vi "Agilent Source and Measure.vi"() -> ()   [LabVIEW 2021]
doc: "Configures the power supply's output range on a channel, configures the DC voltage level, channel appears at the output connector and takes a measurement on the output signal and returns the measured value."
uses:
  <instrlib>/Agilent 3446X Series/Public/Data/Read (Single Point).vi
  <instrlib>/Agilent N6700 Series/Agilent N6700 Series.lvlib
  <instrlib>/Agilent 3446X Series/Agilent 3446X Series.lvlib
panel:
  in  "error in":errorcluster {"code" format="%.0x"}
  out "error out":errorcluster {"code" format="%.0x"}
  out "DMM Voltage Measurement":dbl
  in  "Manual Range":dbl=1.0
  in  "Agilent DMM":refnum<visa-resource-name>
  in  "Absolute Resolution":dbl=1e-06
  in  "Measurement Function":i32(ring)=10 items=["Continuity", "Current AC", "Current DC", "Diode", "Frequency", "Resistance 4-wire", "Period", "Resistance 2-wire", "Temperature", "Voltage AC", "Voltage DC", "Voltage DC Ratio", "Capacitance"]
  in  "Limit":dbl=1.0 format="%^.3e"
  in  "Behavior":i32(ring) items=["Regulatory Limit", "Trip Limit"]
  out "SMU Voltage Measurement":dbl format="%^.3e"
  in  "Voltage Level":dbl=5.0 format="%^.3e"
  in  "Voltage Range":dbl=10.0 format="%^.3e"
  in  "Channel Name":string="1"
  in  "Agilent SMU":refnum<visa-resource-name>
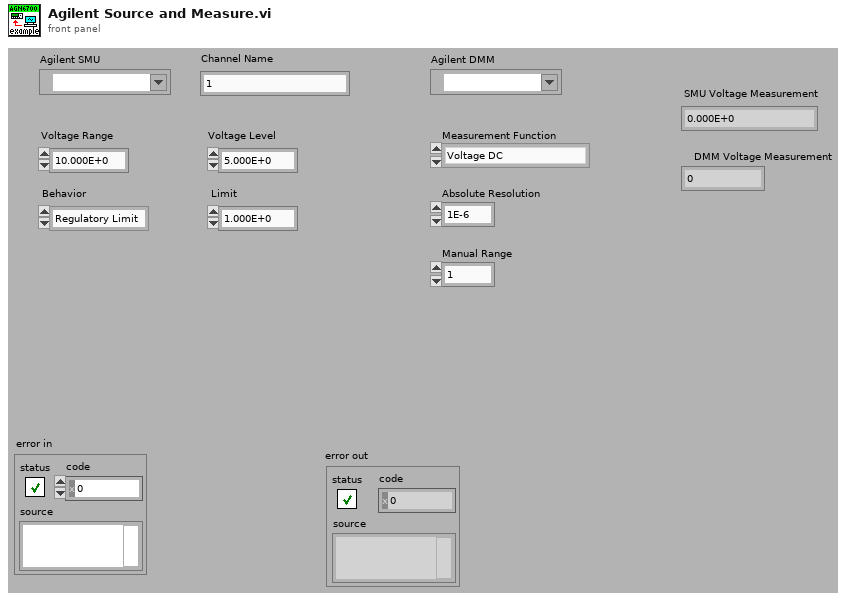
[diagram p1: front panel]
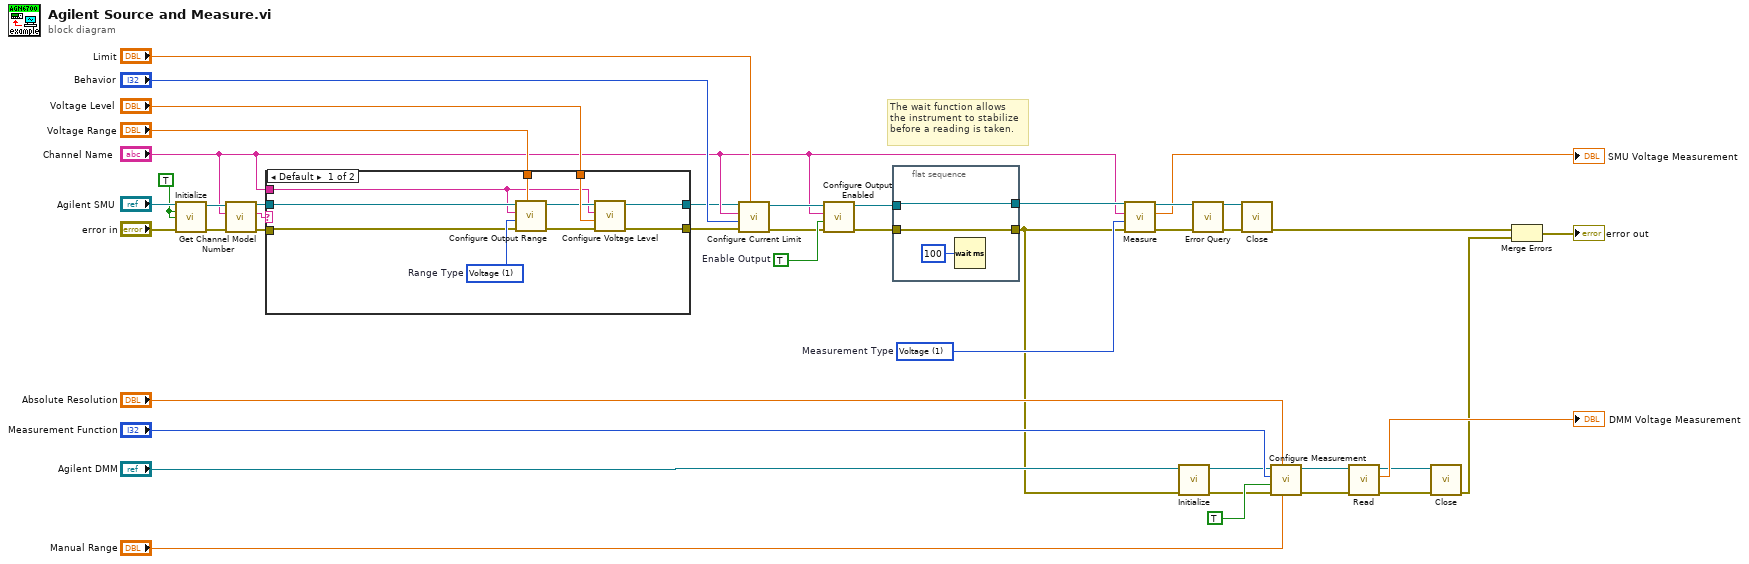
[diagram p0: block diagram]
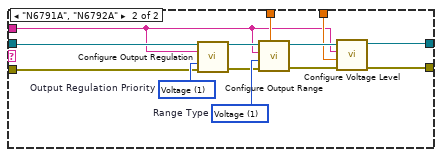
[diagram p2: hidden frame]
diagram:
  w34 = TRUE ("Reset? (T: Yes)")
  w35 = 1 items=["Voltage"=1, "Current"=0]  # Measurement Type
  w36 = TRUE  # Enable Output
  # "The wait function allows \nthe instrument to stabilize\nbefore a reading is taken."
  n1 = call <instrlib>:"Initialize.vi"("VISA resource name"="Agilent SMU", "ID Query? (T: Yes)"=w34, "Reset? (T: Yes)"=w34, "error in (no error)"="error in") -> ("VISA resource name out"=w26:refnum<visa-resource-name>, "error out"=w25:errorcluster)  [unwired: 10 in]
  n2 = call <instrlib>:"Get Channel Model Number.vi"("error in (no error)"=w25, "Channel Name (1)"="Channel Name", "VISA resource name"=w26) -> ("error out"=w23:errorcluster, "Model Number"=w22:string, "VISA resource name out"=w24:refnum<visa-resource-name>)  [unwired: 6 in]
  n3 = case shown="Default" w22 {
    tunnel: "Voltage Range" -> [w50 w66]
    tunnel: "Channel Name" -> [w44 w56]
    tunnel: w24 -> [w52 w61]
    tunnel: w23 -> [w51 w60]
    tunnel: "Voltage Level" -> [w48 w57]
    tunnel: [w46 w54] -> w19
    tunnel: [w45 w55] -> w18
    frame Default {
      w53 = 1 items=["Voltage"=1, "Current"=0]  # Range Type
      n4 = call <instrlib>:"Configure Output Range.vi"("Range (0.0)"=w50, "error in (no error)"=w51, "Range Type (1: Voltage)"=w53, "Channel Name (1)"=w44, "VISA resource name"=w52) -> ("error out"=w49:errorcluster, "VISA resource name out"=w47:refnum<visa-resource-name>)  [unwired: 5 in]
      n5 = call <instrlib>:"Configure Voltage Level.vi"("error in (no error)"=w49, "Level  (0.0 volts)"=w48, "Channel Name (1)"=w44, "VISA resource name"=w47) -> ("error out"=w46:errorcluster, "VISA resource name out"=w45:refnum<visa-resource-name>)  [unwired: 6 in]
    }
    frame "N6791A", "N6792A" {
      w62 = 1 items=["Voltage"=1, "Current"=0]  # Output Regulation Priority
      w65 = 1 items=["Voltage"=1, "Current"=0]  # Range Type
      n6 = call <instrlib>:"Configure Output Regulation.vi"("VISA resource name"=w61, "Channel Name (1)"=w56, "Output Regulation Priority (1: Voltage)"=w62, "error in (no error)"=w60) -> ("VISA resource name out"=w64:refnum<visa-resource-name>, "error out"=w63:errorcluster)  [unwired: 10 in]
      n7 = call <instrlib>:"Configure Output Range.vi"("Range (0.0)"=w66, "error in (no error)"=w63, "Range Type (1: Voltage)"=w65, "Channel Name (1)"=w56, "VISA resource name"=w64) -> ("error out"=w58:errorcluster, "VISA resource name out"=w59:refnum<visa-resource-name>)  [unwired: 5 in]
      n8 = call <instrlib>:"Configure Voltage Level.vi"("error in (no error)"=w58, "Level  (0.0 volts)"=w57, "Channel Name (1)"=w56, "VISA resource name"=w59) -> ("error out"=w54:errorcluster, "VISA resource name out"=w55:refnum<visa-resource-name>)  [unwired: 6 in]
    }
  }
  n9 = call <instrlib>:"Configure Current Limit.vi"("Limit (0.0 amps)"="Limit", "error in (no error)"=w19, "Behavior (0: Regulatory Limit)"="Behavior", "Channel Name (1)"="Channel Name", "VISA resource name"=w18) -> ("error out"=w33:errorcluster, "VISA resource name out"=w32:refnum<visa-resource-name>)  [unwired: 5 in]
  n10 = call <instrlib>:"Configure Output Enabled.vi"("error in (no error)"=w33, "Enable Output (False)"=w36, "Channel Name (1)"="Channel Name", "VISA resource name"=w32) -> ("error out"=w27:errorcluster, "VISA resource name out"=w29:refnum<visa-resource-name>)  [unwired: 6 in]
  n11 = flat-sequence {
    tunnel: w29 -> [w69]
    tunnel: [w69] -> w28
    tunnel: [w67] -> w3
    tunnel: w27 -> [w67]
    frame #0 {
      n12 = Wait (ms)(milliseconds to wait=u32 100) -> ()  [unwired: 1 out]
    }
  }
  n13 = call <instrlib>:"Measure.vi"("error in (no error)"=w3, "Measurement Type (1: Voltage)"=w35, "Channel Name (1)"="Channel Name", "VISA resource name"=w28) -> ("error out"=w43:errorcluster, "Measurement"=→"SMU Voltage Measurement":dbl, "VISA resource name out"=w40:refnum<visa-resource-name>)  [unwired: 5 in]
  n14 = call <instrlib>:"Initialize.vi"("error in (no error)"=w3, "VISA resource name"="Agilent DMM") -> ("error out"=w7:errorcluster, "VISA resource name out"=w6:refnum<visa-resource-name>)  [unwired: 3 in, 5 out]
  n15 = call <instrlib>:"Error Query.vi"("VISA resource name"=w40, "error in (no error)"=w43) -> ("VISA resource name out"=w41:refnum<visa-resource-name>, "error out"=w42:errorcluster)  [unwired: 10 in, 2 out]
  n16 = call <instrlib>:"Close.vi"("VISA resource name"=w41, "error in (no error)"=w42) -> ("error out"=w5:errorcluster)  [unwired: 13 in]
  n17 = call <instrlib>:"Configure Measurement.vi"("Manual Range (1)"="Manual Range", "Absolute Resolution (1E-6)"="Absolute Resolution", "error in (no error)"=w7, "Auto Range (T: Enable)"=TRUE, "Measurement Function (10: Voltage DC)"="Measurement Function", "VISA resource name"=w6) -> ("error out"=w11:errorcluster, "VISA resource name out"=w10:refnum<visa-resource-name>)  [unwired: 4 out]
  n18 = call-poly <instrlib>:"Read.vi"("error in (no error)"=w11, "VISA resource name"=w10) -> ("error out"=w8:errorcluster, "Measurement"=→"DMM Voltage Measurement":dbl, "VISA resource name out"=w9:refnum<visa-resource-name>)  [unwired: 7 out]
  n19 = call <instrlib>:"Close.vi"("error in (no error)"=w8, "VISA resource name"=w9) -> ("error out"=w1:errorcluster)  [unwired: 9 out]
  n20 = Merge Errors(w5, w1) -> (→"error out":errorcluster)
